vi "readInXml.vi"(8 "error in (no error)":errorcluster, 10 "NativeXML out":refnum<class "NativeXML.lvclass">, 11 "deviceDataBase in":refnum<class "deviceDataBase.lvclass">) -> (0 "error out":errorcluster, 3 "deviceDataBase out":refnum<class "deviceDataBase.lvclass">)   [LabVIEW 2011, in "Tools.lvlib" / "DatabaseHelpers.lvlib" / "deviceDataBase.lvclass"]
uses:
  deviceDataBase.lvclass
  NativeXML/NativeXML.lvclass
  deviceDataBase.lvclass/deviceDataBase.ctl
  Database Objects/device/device.lvclass
  Database Objects/DeviceArray/DeviceArray.lvclass
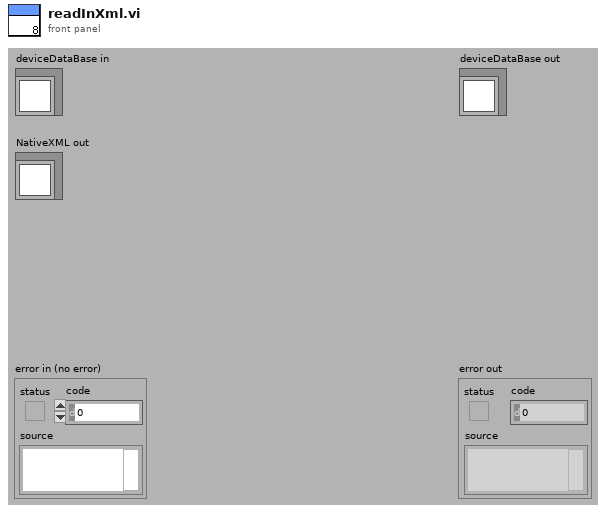
[diagram p1: front panel]
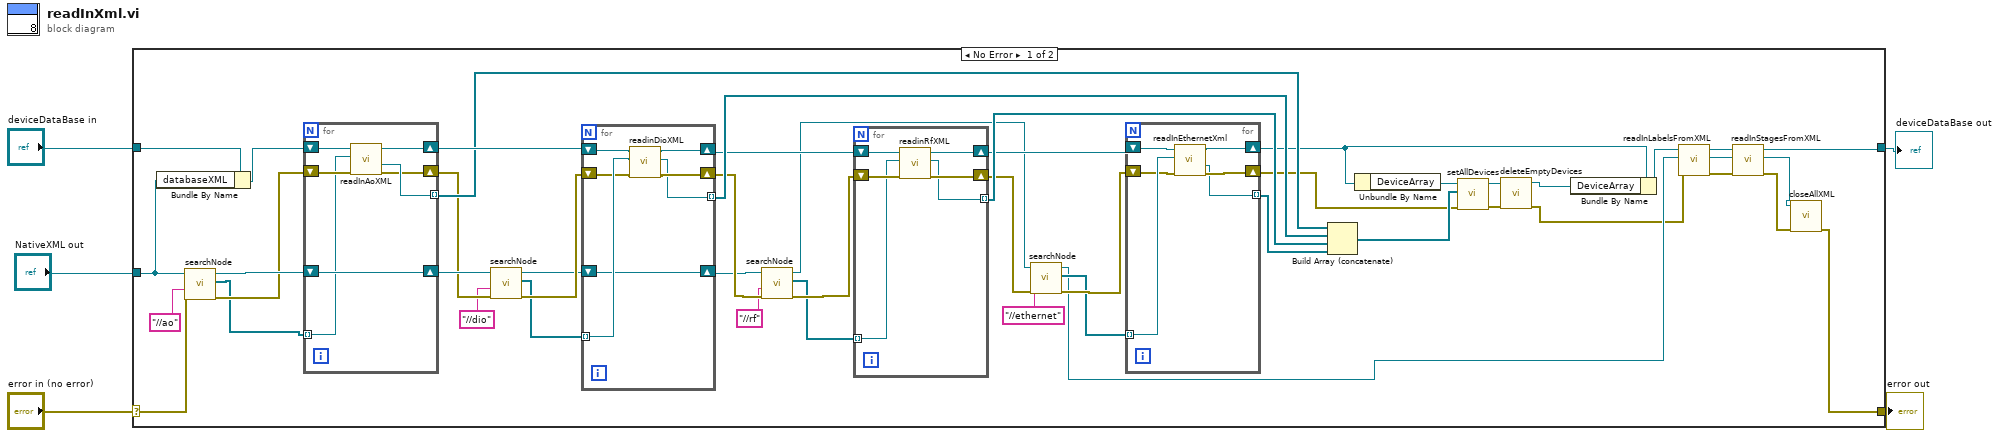
[diagram p0: block diagram]
diagram:
  n1 = case shown="No Error" "error in (no error)" {
    selector: "error in (no error)" -> [w38 w81]
    tunnel: [w12 w81] -> w4
    tunnel: [w7 w80] -> w2
    tunnel: "deviceDataBase in" -> [w53 w80]
    tunnel: "NativeXML out" -> [w35 _]
    frame No Error {
      n2 = Bundle By Name(cluster=w53, "databaseXML"=w35) -> (w52:refnum<class "deviceDataBase.lvclass">)
      n3 = call "searchNode.vi"("error in (no error)"=w38, "searchXPath"="//ao", "NativeXML in"=w35) -> ("error out"=w34:errorcluster, "nodeArray"=w20:refnum<class "NativeXML.lvclass">[], "NativeXML out"=w37:refnum<class "NativeXML.lvclass">)  [unwired: 6 in]
      n4 = for {
        shift-right: [w78] -> w51
        shift-left: w52 -> [w79]
        shift-right: [w74] -> w32
        shift-left: w34 -> [w77]
        tunnel: w20 -> [w73] mode=indexing
        shift-right: [w76] -> w33
        shift-left: w37 -> [w76]
        tunnel: [w75] -> w50 mode=indexing
        n5 = call "readInAoXML.vi"("error in (no error)"=w77, "NativeXML in"=w73, "deviceDataBase in"=w79) -> ("error out"=w74:errorcluster, "device.lvclass out"=w75:refnum<class "device.lvclass">, "deviceDataBase out"=w78:refnum<class "deviceDataBase.lvclass">)  [unwired: 6 in]
      }
      n6 = call "searchNode.vi"("error in (no error)"=w32, "searchXPath"="//dio", "NativeXML in"=w33) -> ("error out"=w30:errorcluster, "nodeArray"=w19:refnum<class "NativeXML.lvclass">[], "NativeXML out"=w29:refnum<class "NativeXML.lvclass">)  [unwired: 6 in]
      n7 = for {
        shift-right: [w71] -> w43
        shift-left: w51 -> [w70]
        shift-right: [w72] -> w27
        shift-left: w30 -> [w68]
        tunnel: w19 -> [w69] mode=indexing
        tunnel: [w67] -> w49 mode=indexing
        shift-right: [w66] -> w26
        shift-left: w29 -> [w66]
        n8 = call "readinDioXML.vi"("error in (no error)"=w68, "channel_configXML"=w69, "deviceDataBase in"=w70) -> ("error out"=w72:errorcluster, "device.lvclass out"=w67:refnum<class "device.lvclass">, "deviceDataBase out"=w71:refnum<class "deviceDataBase.lvclass">)  [unwired: 6 in]
      }
      n9 = call "searchNode.vi"("error in (no error)"=w27, "searchXPath"="//rf", "NativeXML in"=w26) -> ("error out"=w28:errorcluster, "nodeArray"=w18:refnum<class "NativeXML.lvclass">[], "NativeXML out"=w22:refnum<class "NativeXML.lvclass">)  [unwired: 6 in]
      n10 = for {
        shift-right: [w64] -> w41
        shift-left: w43 -> [w65]
        shift-right: [w62] -> w24
        shift-left: w28 -> [w63]
        tunnel: w18 -> [w60] mode=indexing
        tunnel: [w61] -> w42 mode=indexing
        n11 = call "readinRfXML.vi"("error in (no error)"=w63, "xml in"=w60, "deviceDataBase in"=w65) -> ("error out"=w62:errorcluster, "device.lvclass out"=w61:refnum<class "device.lvclass">, "deviceDataBase out"=w64:refnum<class "deviceDataBase.lvclass">)  [unwired: 6 in]
      }
      n12 = call "searchNode.vi"("error in (no error)"=w24, "searchXPath"="//ethernet", "NativeXML in"=w22) -> ("error out"=w25:errorcluster, "nodeArray"=w17:refnum<class "NativeXML.lvclass">[], "NativeXML out"=w14:refnum<class "NativeXML.lvclass">)  [unwired: 6 in]
      n13 = for {
        shift-right: [w58] -> w40
        shift-left: w41 -> [w59]
        shift-right: [w57] -> w16
        shift-left: w25 -> [w54]
        tunnel: w17 -> [w55] mode=indexing
        tunnel: [w56] -> w39 mode=indexing
        n14 = call "readInEthernetXml.vi"("error in (no error)"=w54, "xml in"=w55, "deviceDataBase in"=w59) -> ("error out"=w57:errorcluster, "device.lvclass out"=w56:refnum<class "device.lvclass">, "deviceDataBase out"=w58:refnum<class "deviceDataBase.lvclass">)  [unwired: 6 in]
      }
      n15 = Build Array (concatenate)(w50, w49, w42, w39) -> (w47:refnum<class "device.lvclass">[])
      n16 = Unbundle By Name(w40) -> ("DeviceArray"=w48:refnum<class "DeviceArray.lvclass">)
      n17 = call "setAllDevices.vi"("error in (no error)"=w16, "deviceArray"=w47, "DeviceArray.lvclass in"=w48) -> ("error out"=w46:errorcluster, "DeviceArray.lvclass out"=w45:refnum<class "DeviceArray.lvclass">)  [unwired: 7 in]
      n18 = call "deleteEmptyDevices.vi"("error in (no error)"=w46, "DeviceArray in"=w45) -> ("error out"=w13:errorcluster, "DeviceArray out"=w44:refnum<class "DeviceArray.lvclass">)  [unwired: 8 in]
      n19 = Bundle By Name(cluster=w40, "DeviceArray"=w44) -> (w15:refnum<class "deviceDataBase.lvclass">)
      n20 = call "readInLabelsFromXML.vi"("error in (no error)"=w13, "NativeXML"=w14, "deviceDataBase in"=w15) -> ("error out"=w9:errorcluster, "NativeXML out"=w10:refnum<class "NativeXML.lvclass">, "deviceDataBase out"=w11:refnum<class "deviceDataBase.lvclass">)  [unwired: 6 in]
      n21 = call "readInStagesFromXML.vi"("error in (no error)"=w9, "NativeXML"=w10, "deviceDataBase in"=w11) -> ("error out"=w8:errorcluster, "NativeXML out"=w6:refnum<class "NativeXML.lvclass">, "deviceDataBase out"=w7:refnum<class "deviceDataBase.lvclass">)  [unwired: 6 in]
      n22 = call "closeAllXML.vi"("error in (no error)"=w8, "NativeXML in"=w6) -> ("error out"=w12:errorcluster)  [unwired: 9 in]
    }
    frame Error {
    }
  }
  "error out" <- w4
  "deviceDataBase out" <- w2
